vi "Set Icon Text Error Constant.vi"(8 "error in":errorcluster, 10 "Text":string, 11 "VI in":refnum<vi>) -> (0 "error out":errorcluster, 3 "VI out":refnum<vi>)   [LabVIEW 2020, in "Panther Dashboard.lvlib"]
uses:
  Panther Dashboard.lvlib
  <vilib>/LabVIEW Icon API/API_Text.ctl
  <vilib>/LabVIEW Icon API/lv_icon/Controls/Pathes.ctl
  <vilib>/LabVIEW Icon API/API_User Layer Data.ctl
  <vilib>/Utility/miscctls.llb/LVPoint32TypeDef.ctl
  <vilib>/picture/picture.llb/imagedata.ctl
  <vilib>/LabVIEW Icon API/LabVIEW Icon API.lvlib
  <vilib>/LabVIEW Icon API/lv_icon/lv_icon.lvlib
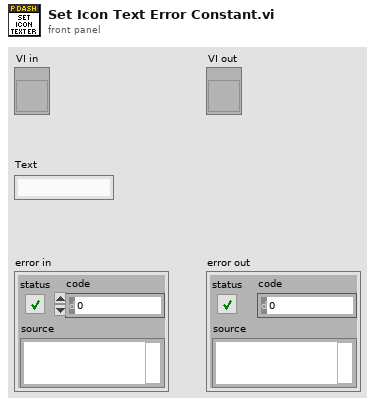
[diagram p1: front panel]
types:
  T1 = typedef "LVPoint32TypeDef.ctl" = cluster{"Horizontal":i32, "Vertical":i32}
  T2 = typedef "LabVIEW Icon API.lvlib/API_User Layer Data.ctl" = cluster{"Layer name":string, "Origin":T1, "Icon image data":T3}
  T3 = typedef "imagedata.ctl" = cluster{"image type":i32, "image depth":i32, "image":u8[], "mask":u8[], "colors":u32[], "Rectangle":cluster{"left":i16, "top":i16, "right":i16, "bottom":i16}}
  T4 = typedef "Pathes.ctl" = enum16{"Root Path", "Icon Templates", "Icon Templates VI", "Icon Templates Lib", "Glyphs"}
  T5 = typedef "LabVIEW Icon API.lvlib/API_Text.ctl" = cluster{"Line 1 text":string, "Line 2 text":string, "Line 3 text":string, "Line 4 text":string}
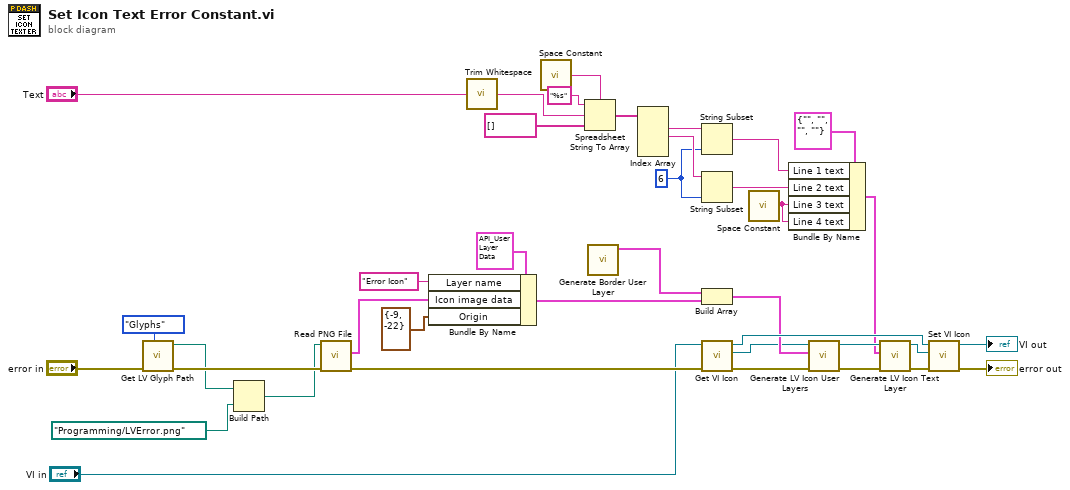
[diagram p0: block diagram]
diagram:
  w18 = 6 ("length (rest)")
  n1 = call <vilib>:"Get LV Glyph Path.vi"("Path"=Pathes."Glyphs", "error in (no error)"="error in") -> ("error out"=w33:errorcluster, "Requested Path"=w16:path)  [unwired: 1 in, 7 out]
  n2 = Build Path(base path=w16, name or relative path=path "Programming/LVError.png") -> (appended path=w2:path)
  n3 = call <vilib>:"Read PNG File.vi"("error in (no error)"=w33, "path to PNG file"=w2) -> ("error out"=w32:errorcluster, "image data"=w12:T3)  [unwired: 7 in, 1 out]
  n4 = Bundle By Name(cluster=T2 {"Layer name"="", "Origin"={"Horizontal"=0, "Vertical"=0}, "Icon image data"={"image type"=0, "image depth"=0, "image"=[], "mask"=[], "colors"=[], "Rectangle"={"left"=0, "top"=0, "right"=0, "bottom"=0}}} ("User layer"), "Layer name"="Error Icon", "Icon image data"=w12, "Origin"=T1 {"Horizontal"=-9, "Vertical"=-22}) -> (w13:T2)
  n5 = call <vilib>:"Trim Whitespace.vi"("string"="Text") -> ("trimmed string"=w29:string)  [unwired: 1 in]
  n6 = call <vilib>:"Space Constant.vi"() -> ("String"=w27:string)
  n7 = Spreadsheet String To Array(delimiter (Tab)=w27, format string="%s", spreadsheet string=w29, array type (2D Dbl)=string[] [] ("format string")) -> (array=w25:string[])
  n8 = call <vilib>:"Generate Border User Layer.vi"() -> ("User Layer data"=w4:T2)  [unwired: 11 in]
  n9 = Index Array(array=w25) -> (element #1=w24:string, element #2=w23:string)  [unwired: 4 in, 2 out]
  n10 = String Subset(string=w24, length (rest)=w18) -> (substring=w22:string)  [unwired: 1 in]
  n11 = String Subset(string=w23, length (rest)=w18) -> (substring=w21:string)  [unwired: 1 in]
  n12 = Build Array(w4, w13) -> (w11:T2[])
  n13 = call <vilib>:"Get VI Icon.vi"("error in (no error)"=w32, "VI Refnum in"="VI in") -> ("error out"=w36:errorcluster, "Icon"=w8:refnum<class "Icon.lvclass">, "VI Refnum out"=w19:refnum<vi>)  [unwired: 7 in]
  n14 = call <vilib>:"Space Constant.vi"() -> ("String"=w3:string)
  n15 = Bundle By Name(cluster=T5 {"Line 1 text"="", "Line 2 text"="", "Line 3 text"="", "Line 4 text"=""} ("Text"), "Line 1 text"=w22, "Line 2 text"=w21, "Line 3 text"=w3, "Line 4 text"=w3) -> (w6:T5)
  n16 = call <vilib>:"Generate LV Icon User Layers.vi"("error in (no error)"=w36, "User layers"=w11, "Icon in"=w8) -> ("error out"=w35:errorcluster, "Icon out"=w9:refnum<class "Icon.lvclass">)  [unwired: 7 in]
  n17 = call <vilib>:"Generate LV Icon Text Layer.vi"("error in (no error)"=w35, "Text"=w6, "Icon in"=w9) -> ("error out"=w34:errorcluster, "Icon out"=w7:refnum<class "Icon.lvclass">)  [unwired: 7 in]
  n18 = call <vilib>:"Set VI Icon.vi"("error in (no error)"=w34, "Icon"=w7, "VI Refnum in"=w19) -> ("error out"=→"error out":errorcluster, "VI Refnum out"=→"VI out":refnum<vi>)  [unwired: 7 in]
